vi "Dynamic Dispatch.vi"() -> ()   [LabVIEW 2011]
uses:
  Classes/Beer.lvclass
  Classes/Ale.lvclass
  Classes/Guiness.lvclass
  Classes/Lager.lvclass
panel:
  in  "Leave":bool
  in  "Pour":bool
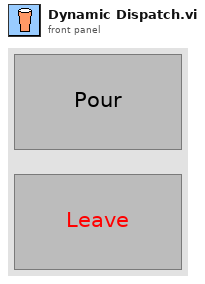
[diagram p1: front panel]
types:
  T1 = enum16{"Left Button", "Center Button", "Right Button", "Window Close"}
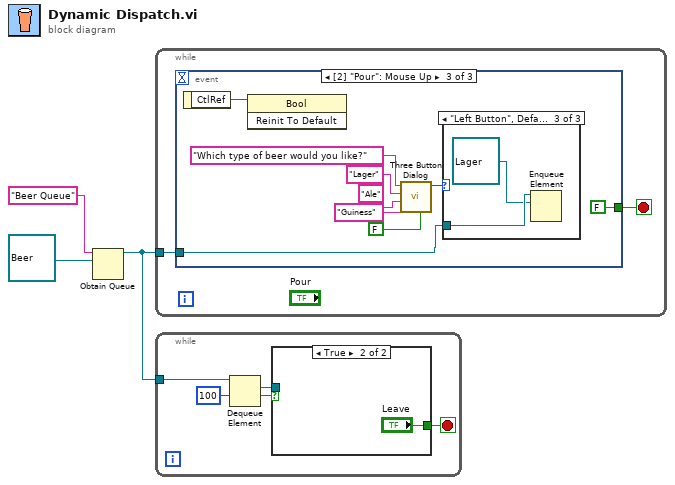
[diagram p0: block diagram]
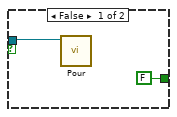
[diagram p2: hidden frame]
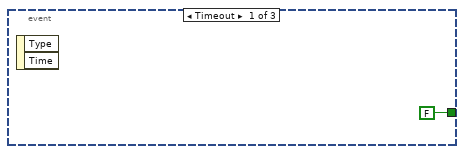
[diagram p3: hidden frame]
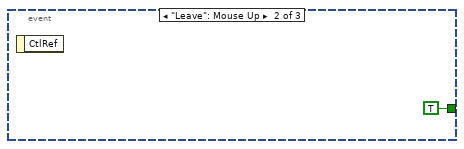
[diagram p4: hidden frame]
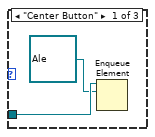
[diagram p5: hidden frame]
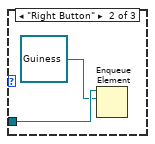
[diagram p6: hidden frame]
diagram:
  n1 = Obtain Queue(name (unnamed)="Beer Queue", element data type=refnum<class "Beer.lvclass"> refnum ("Beer.lvclass")) -> (queue out=w1:refnum<queue>)  [unwired: 3 in, 2 out]
  n2 = while {
    tunnel: w1 -> [w4]
    stop <- w5 stop-if-true
    n3 = event shown="[2] \"Pour\": Mouse Up" {
      selector: _ -> [_ _ _]
      dyn-events: _ -> [_ _ _]
      timeout: _ -> [_ _ _]
      tunnel: [FALSE TRUE FALSE] -> w5
      tunnel: w4 -> [_ _ w8]
      event Timeout {
        n4 = event-data() -> ()  [unwired: 1 in, 2 out]
      }
      event "Leave": Mouse Up {
        n5 = event-data() -> ()  [unwired: 1 in, 1 out]
      }
      event "Pour": Mouse Up {
        n6 = event-data() -> ("CtlRef"=w16:refnum<vi>)  [unwired: 1 in]
        n7 = invoke class="Bool" method="Reinit To Default"(reference=w16) -> ()  [unwired: 2 in, 3 out]
        n8 = call <vilib>:"Three Button Dialog.vi"("Allow user to close window? (TRUE)"=FALSE, "Right Button Text (\"Cancel\")"="Guiness" ("Right Button Text (\"Cancel\")"), "Center Button Text (\"No\")"="Ale" ("Center Button Text (\"No\")"), "Left Button Text (\"Yes\")"="Lager" ("Left Button Text (\"Yes\")"), "message"="Which type of beer would you like?") -> ("Which Button?"=w9:T1)  [unwired: 6 in]
        n9 = case shown="\"Left Button\", Default" w9 {
          tunnel: w8 -> [w18 w20 w22]
          frame "Center Button" {
            n10 = Enqueue Element(queue=w18, element=refnum<class "Ale.lvclass"> refnum ("Ale.lvclass")) -> ()  [unwired: 2 in, 3 out]
          }
          frame "Right Button" {
            n11 = Enqueue Element(queue=w20, element=refnum<class "Guiness.lvclass"> refnum ("Guiness.lvclass")) -> ()  [unwired: 2 in, 3 out]
          }
          frame "Left Button", Default {
            n12 = Enqueue Element(queue=w22, element=refnum<class "Lager.lvclass"> refnum ("Lager.lvclass")) -> ()  [unwired: 2 in, 3 out]
          }
        }
      }
    }
  }
  n13 = while {
    tunnel: w1 -> [w27]
    stop <- w24 stop-if-true
    n14 = Dequeue Element(queue=w27, timeout in ms (-1)=100) -> (element=w23:refnum<class "Beer.lvclass">, timed out?=w25:bool)  [unwired: 1 in, 2 out]
    n15 = case shown="True" w25 {
      tunnel: [FALSE ("Leave") "Leave"] -> w24
      tunnel: w23 -> [w29 _]
      frame False {
        n16 = call-dynamic "Pour.vi"("Beer in"=w29) -> ()  [unwired: 9 in, 2 out]
      }
      frame True {
      }
    }
  }
